vi "Matlab_LoadSequence.vi"() -> ()   [LabVIEW 2015]
panel:
  in  "Quit remote":bool
  out "System SampFreq":dbl
  in  "Cluster":T1={"Volt"=10.0, "frequency probe"=6.0, "Nhemicycles"=8.0, "X0"=0.0, "Foc"=20.0, "Length"=10.0, "NTrig"=10.0, "Prof"=30.0} {"Prof" format="%#_13g"; "NTrig" format="%#_13g"; "Length" format="%#_13g"; "Foc" format="%#_13g"; "X0" format="%#_13g"; "Nhemicycles" format="%#_13g"; "frequency probe" format="%#_13g"; "Volt" format="%#_13g"}
  in  "start sequence":bool
  in  "FOCUSED ELUSEV":T2={"Repeat"=0, "f0 (MHz)"=6.0, "NbHcyble"=1, "focus Z (mm)"=35.0, "Pause Start (us)"=1.0, "X center (mm)"=15.0, "Rx Frequency"=60.0, "Rx center"=0.0, "Pause End (us)"=500.0} {"Pause End (us)" min=0.0; "NbHcyble" min=1 step=1; "Repeat" min=1}
  in  "load sequence":bool
  in  "connect to AIXPLORER":bool
  in  "Stop Button":bool
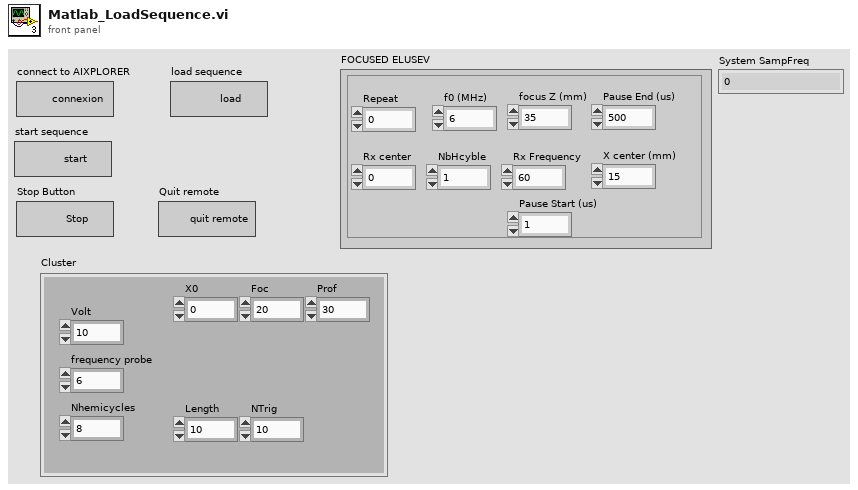
[diagram p1: front panel]
types:
  T1 = cluster{"Volt":dbl, "frequency probe":dbl, "Nhemicycles":dbl, "X0":dbl, "Foc":dbl, "Length":dbl, "NTrig":dbl, "Prof":dbl}
  T2 = cluster{"Repeat":i64, "f0 (MHz)":dbl, "NbHcyble":i64, "focus Z (mm)":dbl, "Pause Start (us)":dbl, "X center (mm)":dbl, "Rx Frequency":dbl, "Rx center":dbl, "Pause End (us)":dbl}
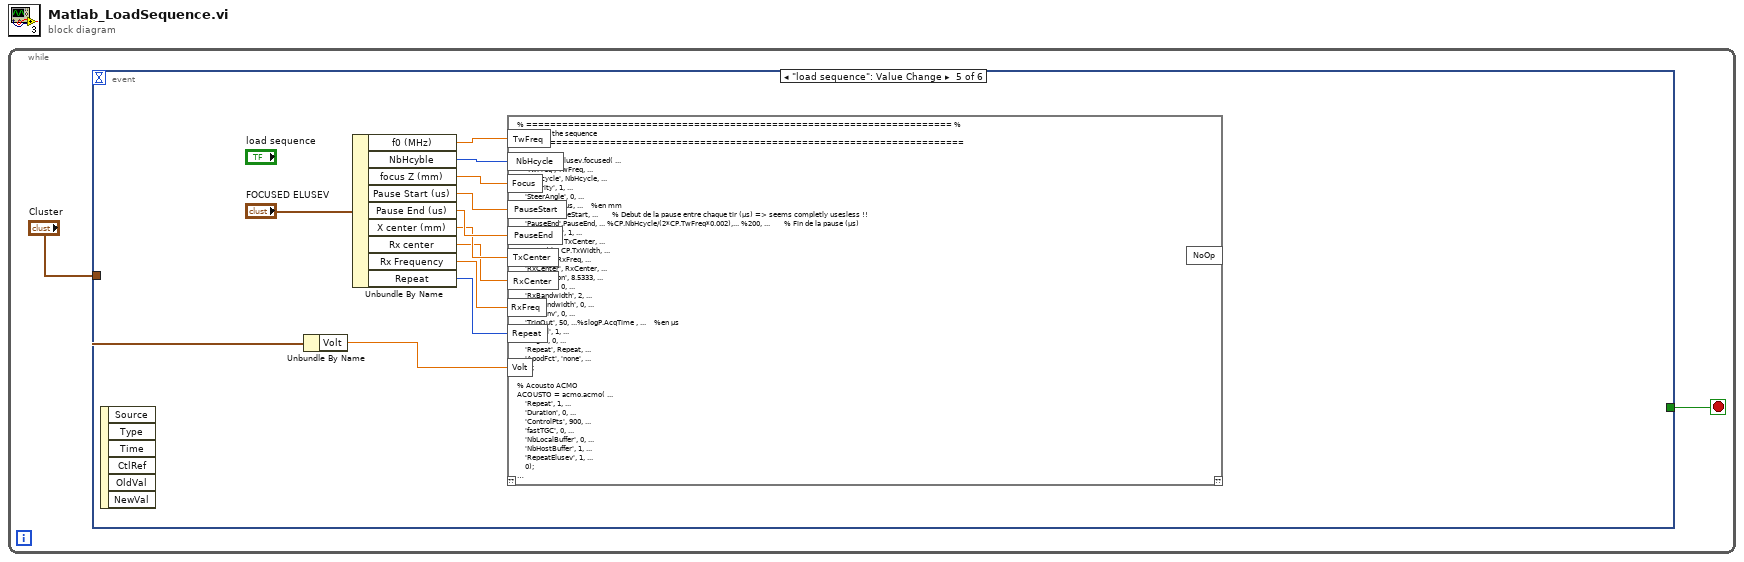
[diagram p0: block diagram]
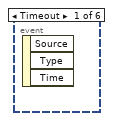
[diagram p2: hidden frame]
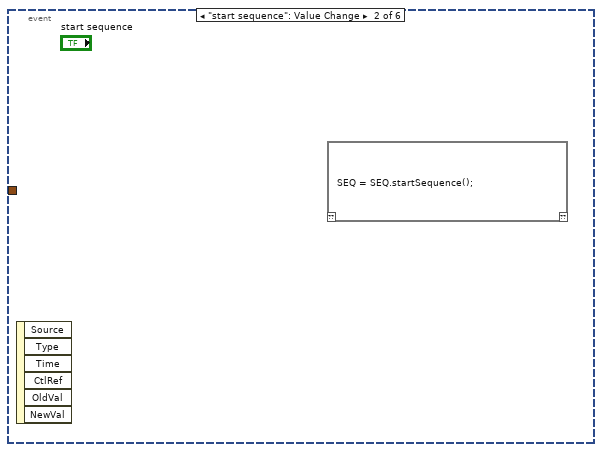
[diagram p3: hidden frame]
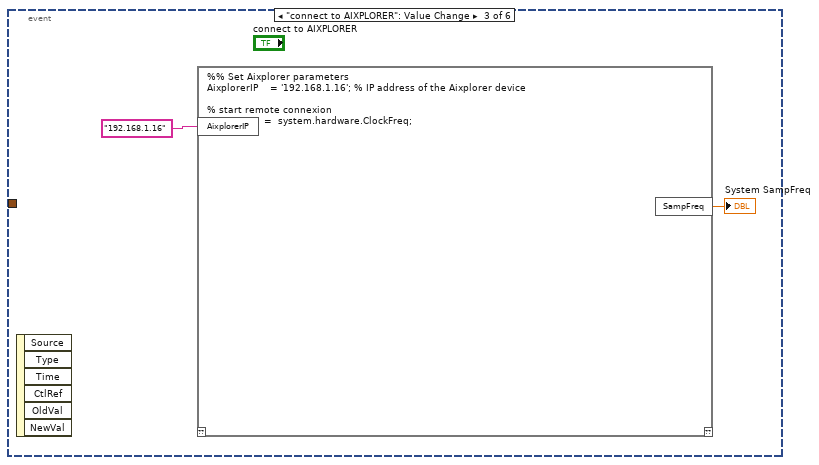
[diagram p4: hidden frame]
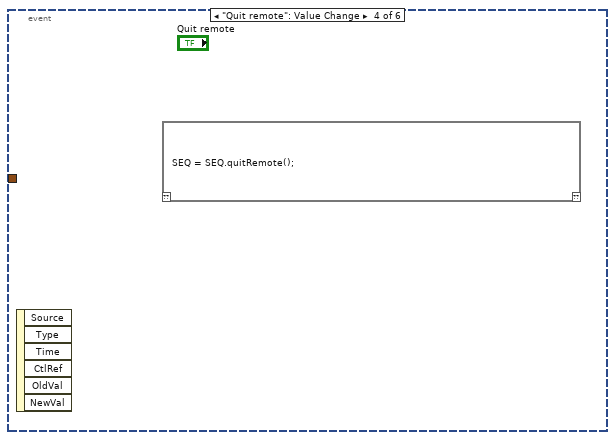
[diagram p5: hidden frame]
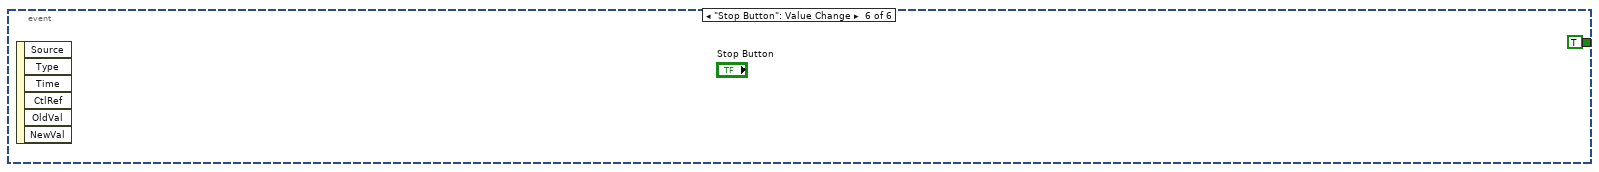
[diagram p6: hidden frame]
diagram:
  n1 = while {
    stop <- w2 stop-if-true
    n2 = event shown="[4] \"load sequence\": Value Change" {
      selector: _ -> [_ _ _ _ _ _]
      dyn-events: _ -> [_ _ _ _ _ _]
      timeout: _ -> [_ _ _ _ _ _]
      tunnel: [_ _ _ _ _ TRUE ("Stop Button")] -> w2
      tunnel: "Cluster" -> [_ _ _ _ w6 _]
      event Timeout {
        n3 = event-data() -> ()  [unwired: 1 in, 3 out]
      }
      event "start sequence": Value Change {
        n4 = event-data() -> ()  [unwired: 1 in, 6 out]
        n5 = script code="SEQ = SEQ.startSequence();"() -> ()  [unwired: 1 in, 1 out]
      }
      event "connect to AIXPLORER": Value Change {
        n6 = event-data() -> ()  [unwired: 1 in, 6 out]
        n7 = script code="%% Set Aixplorer parameters\nAixplorerIP    = '192.168.1.16'; % IP address of the Aixplorer device\n\n% start remote connexion\nSampFreq   =  system.hardware.ClockFreq;"("AixplorerIP"="192.168.1.16" ("String")) -> ("SampFreq"=→"System SampFreq":dbl)  [unwired: 1 in, 1 out]
      }
      event "Quit remote": Value Change {
        n8 = event-data() -> ()  [unwired: 1 in, 6 out]
        n9 = script code="SEQ = SEQ.quitRemote();"() -> ()  [unwired: 1 in, 1 out]
      }
      event "load sequence": Value Change {
        n10 = event-data() -> ()  [unwired: 1 in, 6 out]
        n11 = Unbundle By Name(w6) -> ("Volt"=w5:dbl)
        n12 = Unbundle By Name("FOCUSED ELUSEV") -> ("f0 (MHz)"=w15:dbl, "NbHcyble"=w14:i64, "focus Z (mm)"=w13:dbl, "Pause Start (us)"=w12:dbl, "Pause End (us)"=w11:dbl, "X center (mm)"=w10:dbl, "Rx center"=w9:dbl, "Rx Frequency"=w8:dbl, "Repeat"=w7:i64)
        n13 = script code="% ======================================================================= %\n%% Build the sequence\n% =========================================================================\n\nFOCUSED = elusev.focused( ...\n    'TwFreq', TwFreq, ...\n    'NbHcycle', NbHcycle, ...\n    'Polarity', 1, ...\n    'SteerAngle', 0, ...\n    'Focus', Focus, ...    %en mm\n    'Pause',PauseStart, ...       % Debut de la pause entre chaque tir (µs) => seems completly usesless !!\n    'PauseEnd',PauseEnd, ... %CP.NbHcycle/(2*CP.TwFreq*0.002),... %200, ...       % Fin de la pause (µs)\n    'DutyCycle', 1, ...\n    'TxCenter', TxCenter, ...\n    'TxWidth', CP.TxWidth, ...\n    'RxFreq', RxFreq, ...\n    'RxCenter', RxCenter, ...\n    'RxDuration', 8.5333, ...\n    'RxDelay', 0, ...\n    'RxBandwidth', 2, ...\n    'FIRBandwidth', 0, ...\n    'PulseInv', 0, ...\n    'TrigOut', 50, ...%slogP.AcqTime , ...    %en µs\n    'TrigAll', 1, ...\n    'TrigIn', 0, ...\n    'Repeat', Repeat, ...\n    'ApodFct', 'none', ...\n    0);\n\n% Acousto ACMO\nACOUSTO = acmo.acmo( ...\n    'Repeat', 1, ...\n    'Duration', 0, ...\n    'ControlPts', 900, ...\n    'fastTGC', 0, ...\n    'NbLocalBuffer', 0, ...\n    'NbHostBuffer', 1, ...\n    'RepeatElusev', 1, ...\n    0);\n\nACOUSTO = ACOUSTO.setParam('elusev',FOCUSED,'Ordering',[1]);\n\nclear 'FOCUSED'\n\n% ============================================================================ %\n\n% Create sequence\nTPC = remote.tpc( ...\n    'imgVoltage',Volt, ...\n    'imgCurrent', 0.1, ...\n    'pushVoltage', 25, ...\n    'pushCurrent', 5, ...\n    0);\nSEQ = usse.usse( ...\n    'TPC', TPC, ...\n    'acmo', ACOUSTO, ...\n    'Repeat', 1, ...\n    'Loop', 0, ...\n    'DropFrames', 0, ...\n    0);\n\nclear 'ACOUSTO'\nclear 'TPC'\n\n% Build the REMOTE structur\n[SEQ NbAcq] = SEQ.buildRemote();\nSEQ = SEQ.initializeRemote('IPaddress', AixplorerIP);\nSEQ = SEQ.loadSequence();"("TwFreq"=w15, "NbHcycle"=w14, "Focus"=w13, "PauseStart"=w12, "PauseEnd"=w11, "TxCenter"=w10, "RxCenter"=w9, "RxFreq"=w8, "Repeat"=w7, "Volt"=w5) -> ()  [unwired: 1 in, 2 out]
      }
      event "Stop Button": Value Change {
        n14 = event-data() -> ()  [unwired: 1 in, 6 out]
      }
    }
  }
